vi "CAL_GCP_R.vi"(0 "Initialize":bool, 5 "R_ROLL":sgl, 7 "출력 클러스터 2":T1, 9 "B_ACC":sgl, 11 "R_power_raw":sgl) -> (3 "R_power_OK":bool, 4 "R_Ctrl_Start":bool, 6 "R_GCP":sgl, 8 "출력 클러스터":T1, 10 "R_Period":sgl, 15 "CAN":enum16{"stand", "init", "read"}(ring))   [LabVIEW 2019]
panel:
  out "R_power":sgl[](array[numeric])
  out "R_Run_OK":bool
  out "R_NUM":u32
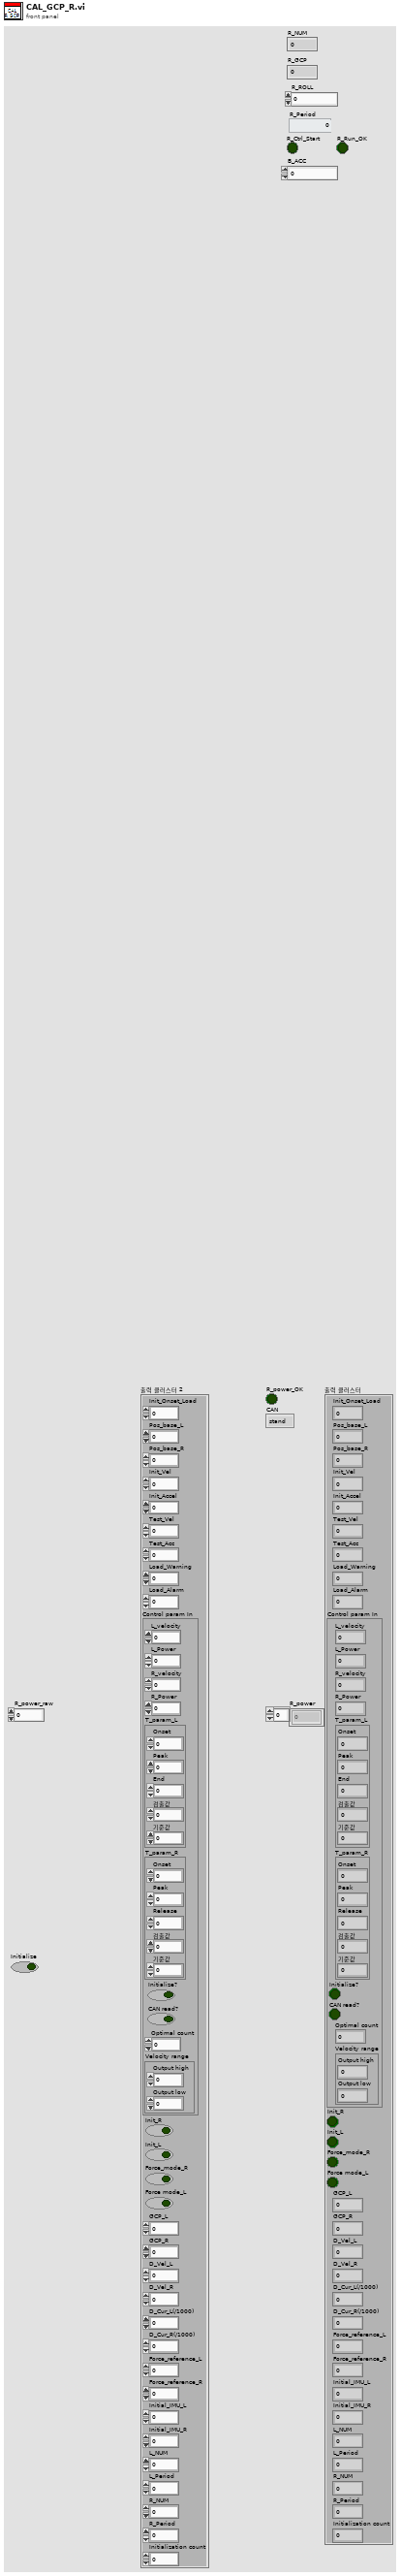
[diagram p1: front panel]
types:
  T1 = cluster{"Init_Onset_Load":sgl, "Pos_base_L":sgl, "Pos_base_R":sgl, "Init_Vel":i32, "Init_Accel":u32, "Test_Vel":i32, "Test_Acc":u32, "Load_Warning":sgl, "Load_Alarm":sgl, "Control param In":cluster{"L_velocity":u32, "L_Power":sgl, "R_velocity":u32, "R_Power":sgl, "T_param_L":cluster{"Onset":sgl, "Peak":sgl, "End":sgl, "검출값":sgl, "기준값":sgl}, "T_param_R":cluster{"Onset":sgl, "Peak":sgl, "Release":sgl, "검출값":sgl, "기준값":sgl}, "Initialize?":bool, "CAN read?":bool, "Optimal count":i32, "Velocity range":cluster{"Output high":dbl, "Output low":dbl}}, "Init_R":bool, "Init_L":bool, "Force_mode_R":bool, "Force mode_L":bool, "GCP_L":sgl, "GCP_R":sgl, "D_Vel_L":sgl, "D_Vel_R":sgl, "D_Cur_L(/1000)":sgl, "D_Cur_R(/1000)":sgl, "Force_reference_L":sgl, "Force_reference_R":sgl, "Initial_IMU_L":sgl, "Initial_IMU_R":sgl, "L_NUM":u32, "L_Period":i16, "R_NUM":u32, "R_Period":i16, "Initialization count":i32}
  T2 = enum16{"Init", "HF", "Cross", "HE", "Cross_E", "Init_F"}
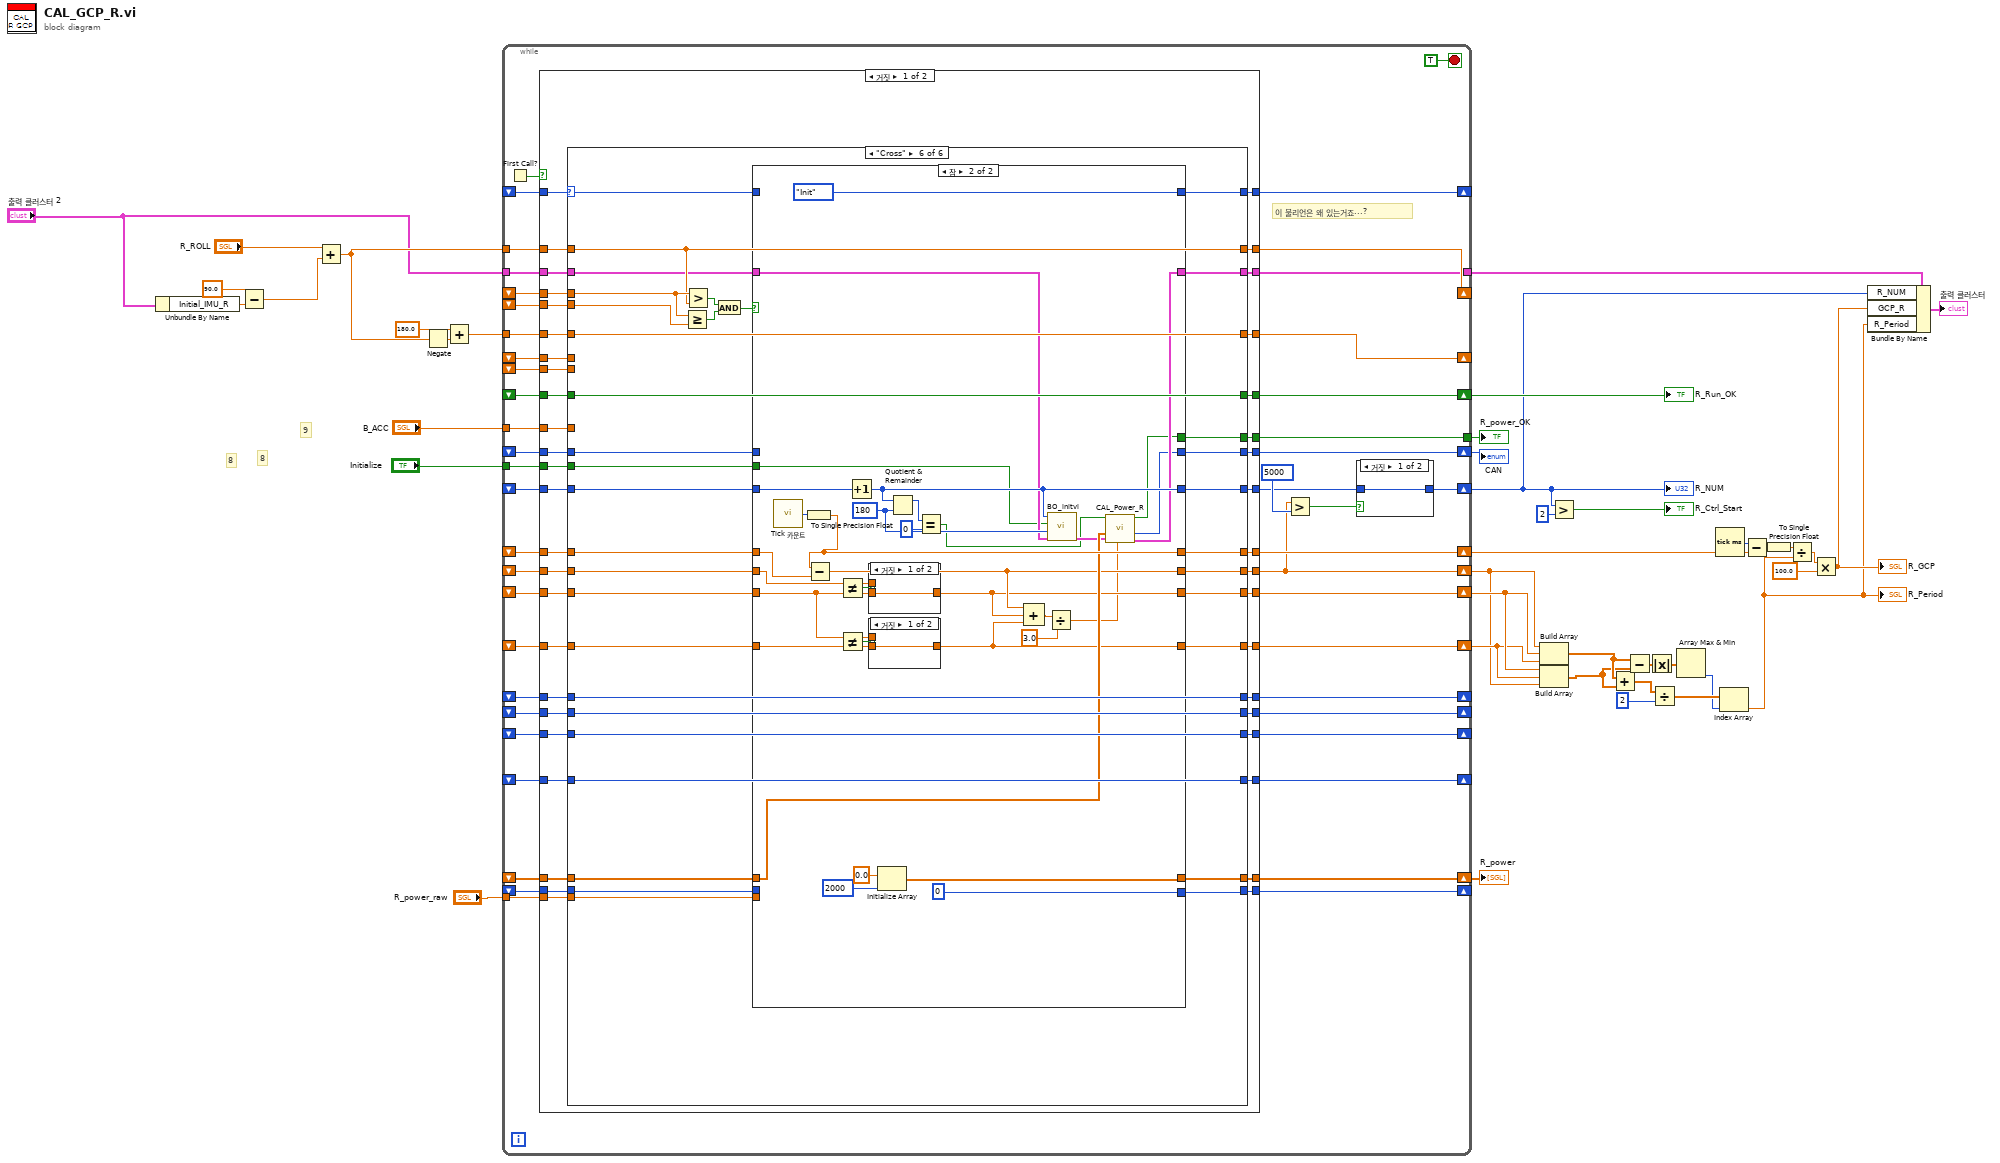
[diagram p0: block diagram]
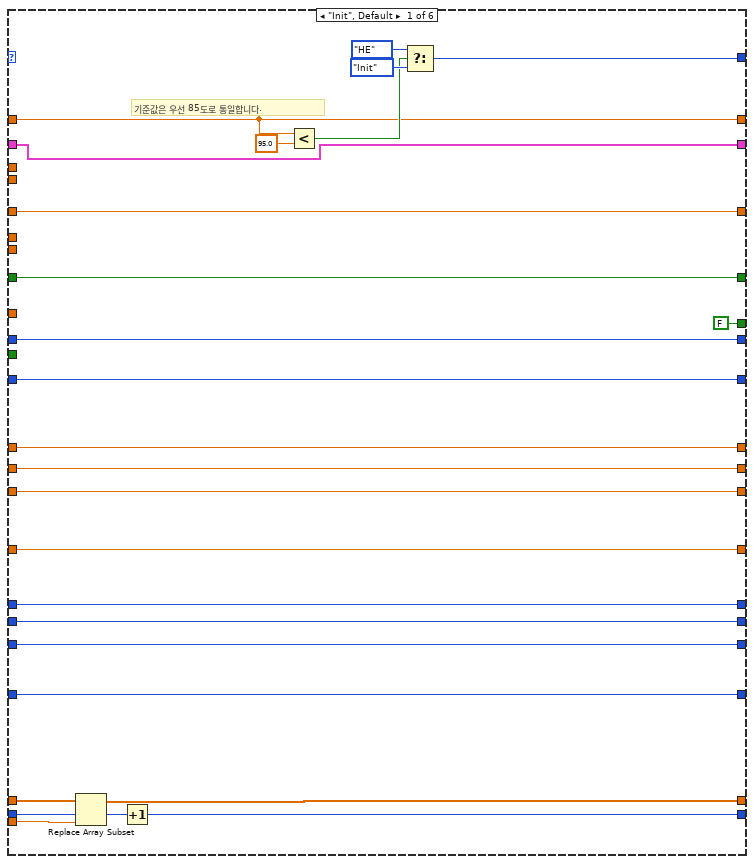
[diagram p2: hidden frame]
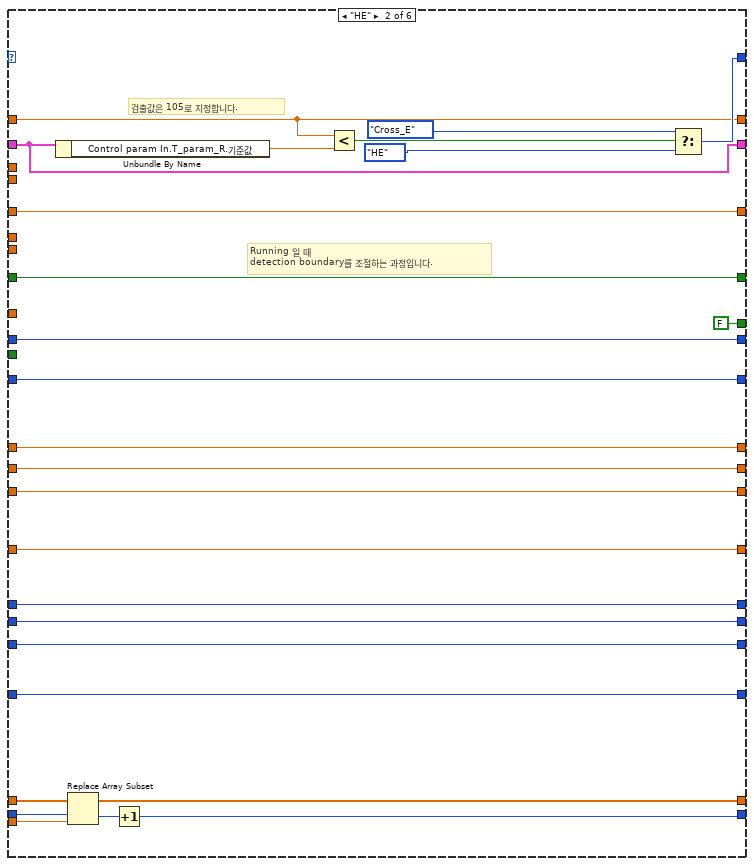
[diagram p3: hidden frame]
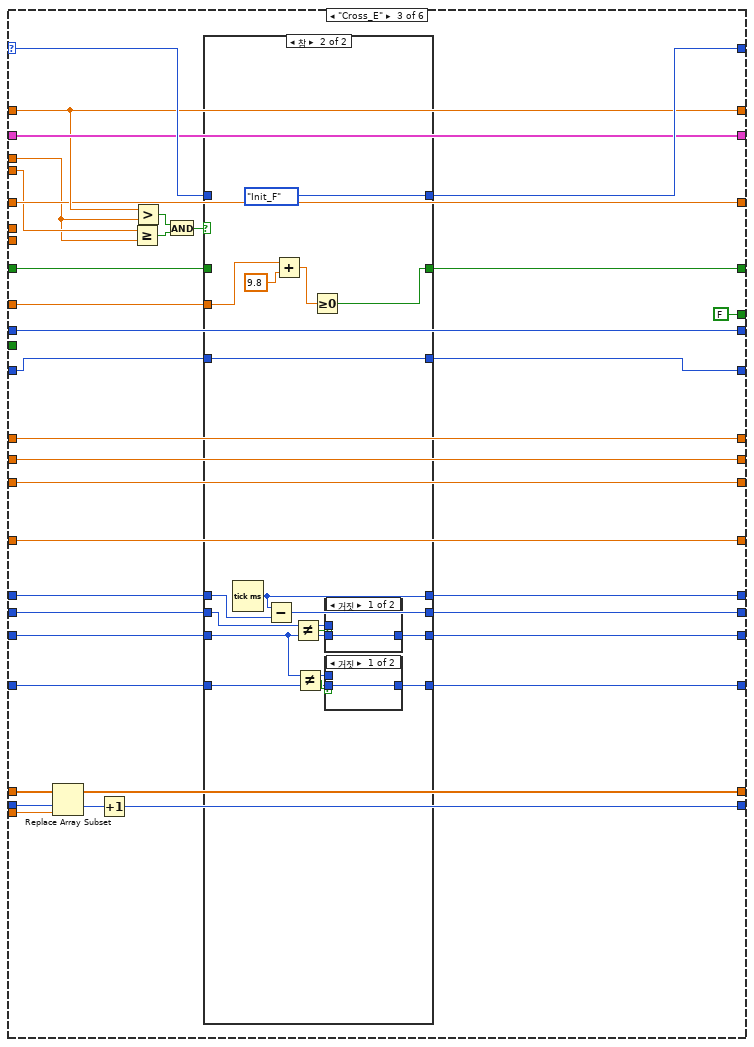
[diagram p4: hidden frame]
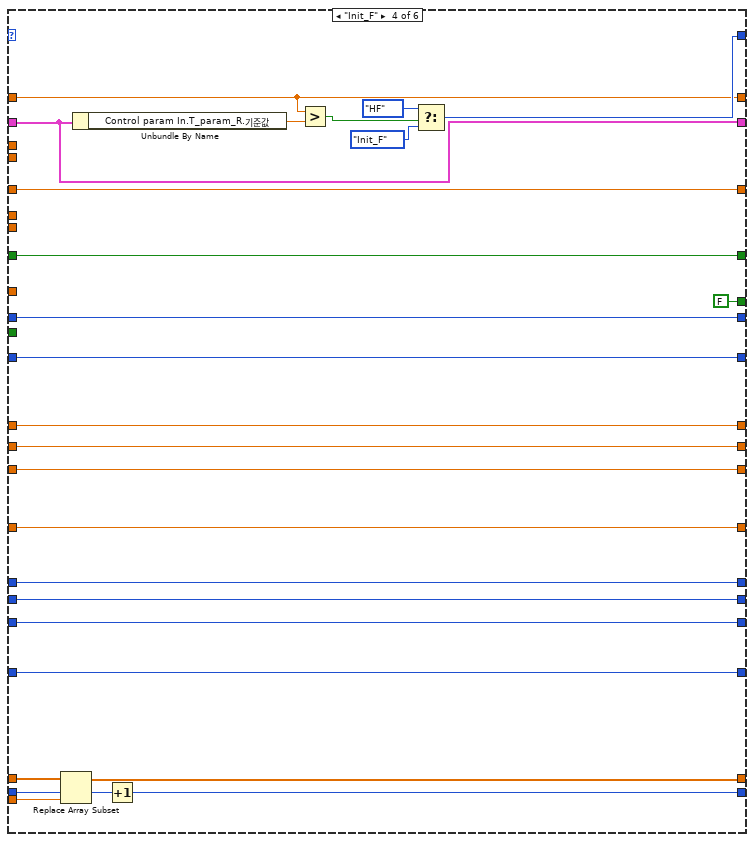
[diagram p8: hidden frame]
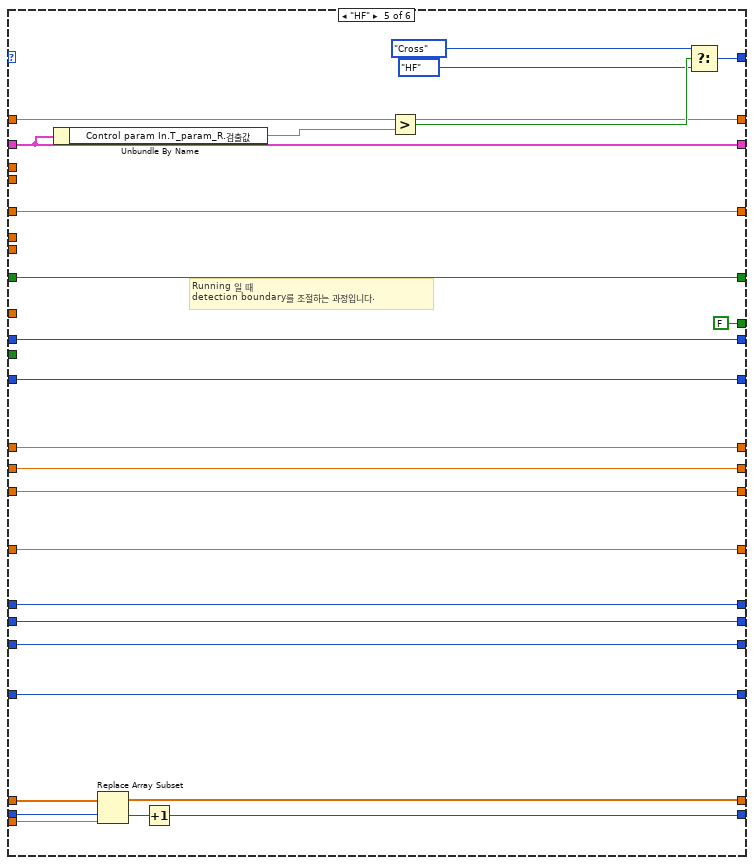
[diagram p9: hidden frame]
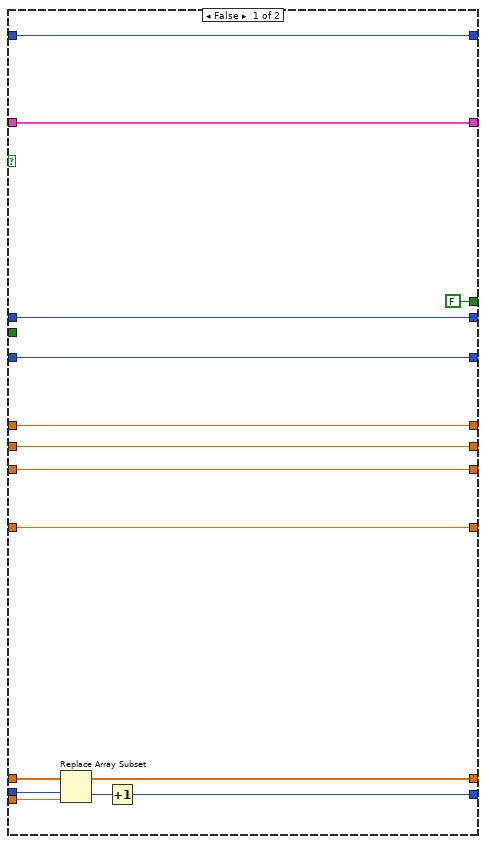
[diagram p10: hidden frame]
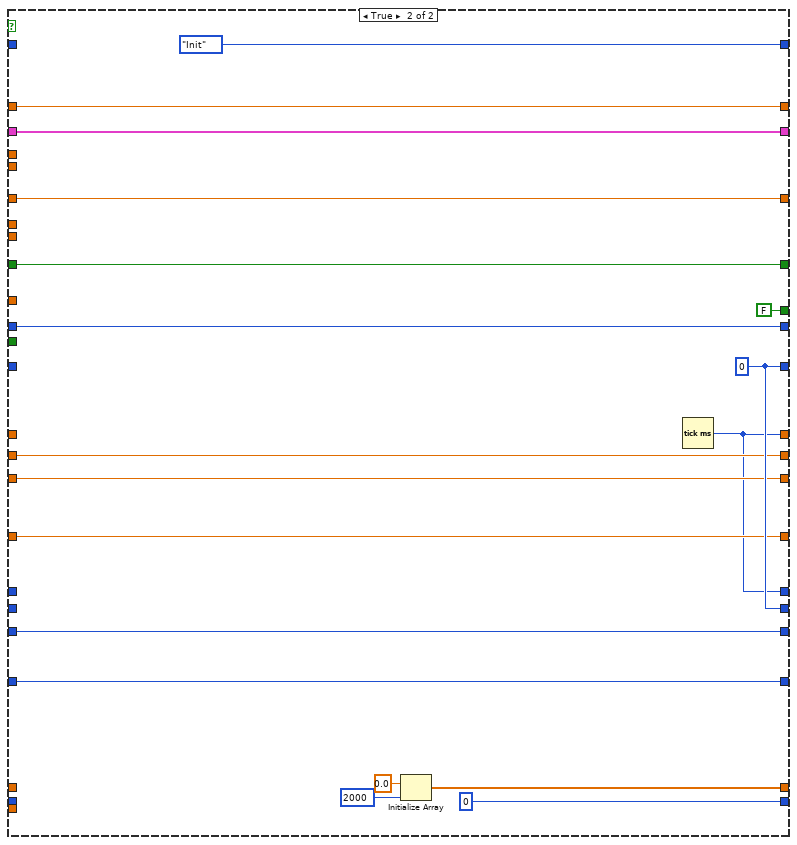
[diagram p13: hidden frame]
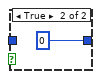
[diagram p14: hidden frame]
diagram:
  # "8"
  # "8"
  # "9"
  n1 = Unbundle By Name("출력 클러스터 2") -> ("Initial_IMU_R"=w5:sgl)
  n2 = Subtract(x=sgl 90.0, y=w5) -> (x-y=w1:sgl)
  n3 = Add(x="R_ROLL", y=w1) -> (x+y=w15:sgl)
  n4 = Negate(x=w15) -> (-x=w33:sgl)
  n5 = Add(x=sgl 180.0, y=w33) -> (x+y=w30:sgl)
  n6 = while {
    tunnel: w15 -> [w84]
    tunnel: "출력 클러스터 2" -> [w81]
    shift-right: [w53] -> _
    shift-left: _ -> [w52]
    shift-right: [w85] -> _
    shift-left: _ -> [w80]
    shift-left: _ -> [w79]
    shift-right: [w76] -> w11
    shift-left: _ -> [w83]
    shift-right: [w66] -> _
    shift-left: _ -> [w82]
    tunnel: w30 -> [w74]
    shift-right: [w73] -> _
    shift-left: _ -> [w72]
    shift-left: _ -> [w71]
    shift-right: [w70] -> w29
    shift-left: _ -> [w69]
    tunnel: "B_ACC" -> [w68]
    shift-right: [w65] -> _
    shift-left: _ -> [w67]
    shift-right: [w58] -> w22
    shift-left: _ -> [w57]
    shift-right: [w55] -> w21
    shift-left: _ -> [w56]
    shift-right: [w64] -> _
    shift-left: _ -> [w63]
    shift-right: [w61] -> _
    shift-left: _ -> [w62]
    shift-right: [w60] -> w28
    shift-left: _ -> [w59]
    shift-right: [w51] -> w20
    shift-left: _ -> [w54]
    shift-right: [w50] -> w13
    shift-left: _ -> [w48]
    shift-right: [w49] -> _
    shift-left: _ -> [w47]
    tunnel: "R_power_raw" -> [w46]
    tunnel: [w45] -> w12
    tunnel: "Initialize" -> [w44]
    tunnel: [w43] -> w7
    shift-right: [w42] -> w6
    shift-left: _ -> [w41]
    stop <- TRUE stop-if-true
    # "이 불리언은 왜 있는거죠...?"
    n7 = First Call?() -> (First Call?: T/F=w86:bool)
    n8 = case shown="거짓" w86 {
      tunnel: [w127 w393] -> w85
      tunnel: w84 -> [w128 w393]
      tunnel: w83 -> [w125 _]
      tunnel: [w126 w392] -> w75
      tunnel: [w123 w383] -> w66
      tunnel: [w122 w392] -> w65
      tunnel: w82 -> [w124 _]
      tunnel: w81 -> [w129 w378]
      tunnel: w80 -> [w121 _]
      tunnel: w79 -> [w120 _]
      tunnel: w74 -> [w119 w391]
      tunnel: [w118 w391] -> w73
      tunnel: w72 -> [w117 _]
      tunnel: w71 -> [w116 _]
      tunnel: [w114 w390] -> w70
      tunnel: w69 -> [w115 w390]
      tunnel: w68 -> [w113 _]
      tunnel: w67 -> [w112 _]
      tunnel: [w111 w389] -> w64
      tunnel: w63 -> [w110 w389]
      tunnel: w62 -> [w109 w388]
      tunnel: [w108 w388] -> w61
      tunnel: [w107 w383] -> w60
      tunnel: w59 -> [w106 _]
      tunnel: [w105 w387] -> w58
      tunnel: w57 -> [w104 w387]
      tunnel: w56 -> [w103 w386]
      tunnel: [w102 w386] -> w55
      tunnel: [w101 w385] -> w51
      tunnel: w54 -> [w100 w385]
      tunnel: [w98 T2."Init"] -> w53
      tunnel: w52 -> [w99 _]
      tunnel: [w94 w380] -> w50
      tunnel: [w93 0] -> w49
      tunnel: w48 -> [w97 _]
      tunnel: w47 -> [w96 _]
      tunnel: w46 -> [w95 _]
      tunnel: [w92 w378] -> w45
      tunnel: w44 -> [w91 _]
      tunnel: [w90 FALSE ("R_power_OK")] -> w43
      tunnel: [w89 w376] -> w42
      tunnel: w41 -> [w88 w376]
      frame False {
        n9 = case shown="\"Cross\"" w99 {
          selector: w99 -> [_ _ w213 _ _ w325]
          tunnel: w129 -> [w133 w158 w186 w241 w270 w296]
          tunnel: w128 -> [w131 w155 w183 w261 w289 w318]
          tunnel: [w131 w155 w183 w261 w289 w318] -> w127
          tunnel: [w154 w178 w211 w258 w288 w320] -> w126
          tunnel: w125 -> [w154 w178 w212 w258 w288 w321]
          tunnel: w124 -> [w153 w177 w209 w257 w287 w313]
          tunnel: [w153 w177 w210 w257 w287 w313] -> w123
          tunnel: [w150 w176 w208 w256 w286 w316] -> w122
          tunnel: w121 -> [_ _ w180 _ _ w319]
          tunnel: w120 -> [_ _ w181 _ _ w324]
          tunnel: w119 -> [w152 w172 w182 w260 w282 w310]
          tunnel: [w152 w172 w182 w260 w282 w310] -> w118
          tunnel: w117 -> [_ _ _ _ _ _]
          tunnel: w116 -> [_ _ _ _ _ _]
          tunnel: w115 -> [w151 w169 w207 w259 w267 w309]
          tunnel: [w151 w169 w206 w259 w267 w309] -> w114
          tunnel: w113 -> [_ _ w205 _ _ _]
          tunnel: w112 -> [w150 w176 w193 w256 w286 w316]
          tunnel: [w149 w175 w201 w254 w285 w315] -> w111
          tunnel: w110 -> [w149 w175 w192 w254 w285 w315]
          tunnel: w109 -> [w148 w174 w200 w253 w284 w314]
          tunnel: [w148 w174 w199 w253 w284 w314] -> w108
          tunnel: [w147 w173 w198 w255 w283 w312] -> w107
          tunnel: w106 -> [w147 w173 w198 w255 w283 w311]
          tunnel: [w146 w171 w196 w251 w281 w308] -> w105
          tunnel: w104 -> [w146 w171 w196 w251 w281 w307]
          tunnel: w103 -> [w145 w170 w197 w250 w280 w306]
          tunnel: [w145 w170 w197 w250 w280 w305] -> w102
          tunnel: [w144 w168 w195 w252 w279 w304] -> w101
          tunnel: w100 -> [w144 w168 w195 w252 w279 w303]
          tunnel: [w143 w165 w194 w262 w276 w302] -> w98
          tunnel: w97 -> [w139 w164 w191 w248 w275 w301]
          tunnel: w96 -> [w136 w163 w190 w247 w274 w300]
          tunnel: w95 -> [w138 w162 w189 w246 w273 w299]
          tunnel: [w137 w161 w187 w245 w272 w297] -> w94
          tunnel: [w135 w160 w188 w244 w271 w298] -> w93
          tunnel: [w133 w158 w186 w241 w270 w295] -> w92
          tunnel: w91 -> [_ _ _ _ _ w294]
          tunnel: [FALSE ("R_power_OK") FALSE ("R_power_OK") FALSE ("R_power_OK") FALSE ("R_power_OK") FALSE ("R_power_OK") w293] -> w90
          tunnel: [w132 w157 w184 w242 w268 w292] -> w89
          tunnel: w88 -> [w132 w157 w184 w242 w268 w291]
          frame "Init", Default {
            # "기준값은 우선 85도로 통일합니다."
            n10 = Replace Array Subset(array=w139, new element=w138, index=w136) -> (w137:sgl[])
            n11 = Increment(x=w136) -> (x+1=w135:i32)
            n12 = Less?(x=w131, y=sgl 95.0) -> (x < y?=w140:bool)
            n13 = Select(t=T2."HE", s=w140, f=T2."Init") -> (s? t:f=w143:T2)
          }
          frame "HE" {
            # "Running 일 때 \ndetection boundary를 조절하는 과정입니다."
            # "검출값은 105로 지정합니다."
            n14 = Unbundle By Name(w158) -> ("Control param In.T_param_R.기준값"=w156:sgl)
            n15 = Replace Array Subset(array=w164, new element=w162, index=w163) -> (w161:sgl[])
            n16 = Increment(x=w163) -> (x+1=w160:i32)
            n17 = Less?(x=w155, y=w156) -> (x < y?=w179:bool)
            n18 = Select(t=T2."Cross_E", s=w179, f=T2."HE") -> (s? t:f=w165:T2)
          }
          frame "Cross_E" {
            n19 = Replace Array Subset(array=w191, new element=w189, index=w190) -> (w187:sgl[])
            n20 = Increment(x=w190) -> (x+1=w188:i32)
            n21 = Greater Or Equal?(x=w181, y=w180) -> (x >= y?=w204:bool)
            n22 = Greater?(x=w183, y=w180) -> (0:w203:bool)
            n23 = And(x=w203, y=w204) -> (x .and. y?=w202:bool)
            n24 = case shown="참" w202 {
              tunnel: w213 -> [w218 _]
              tunnel: [w218 T2."Init_F"] -> w194
              tunnel: w212 -> [w219 w227]
              tunnel: [w219 w227] -> w211
              tunnel: w209 -> [w220 w236]
              tunnel: [w215 w226] -> w208
              tunnel: [w220 w235] -> w210
              tunnel: w207 -> [w217 _]
              tunnel: [w217 w232] -> w206
              tunnel: w205 -> [_ w221]
              tunnel: [w214 w231] -> w201
              tunnel: w200 -> [w216 w230]
              tunnel: [w216 w229] -> w199
              tunnel: w193 -> [w215 w225]
              tunnel: w192 -> [w214 w224]
              frame False {
              }
              frame True {
                n25 = Tick Count (ms)() -> (millisecond timer value=w235:u32)
                n26 = Subtract(x=w235, y=w236) -> (x-y=w226:u32)
                n27 = Add(x=w221, y=9.8) -> (x+y=w222:dbl)
                n28 = Not Equal?(x=w225, y=w224) -> (x != y?=w234:bool)
                n29 = Not Equal?(x=w224, y=w230) -> (x != y?=w233:bool)
                n30 = Greater Or Equal To 0?(x=w222) -> (x >= 0?=w232:bool)
                n31 = case shown="거짓" w234 {
                  tunnel: [w239 w240] -> w231
                  tunnel: w225 -> [_ w240]
                  tunnel: w224 -> [w239 _]
                  frame False {
                  }
                  frame True {
                  }
                }
                n32 = case shown="거짓" w233 {
                  tunnel: w224 -> [_ w238]
                  tunnel: w230 -> [w237 _]
                  tunnel: [w237 w238] -> w229
                  frame False {
                  }
                  frame True {
                  }
                }
              }
            }
          }
          frame "Init_F" {
            n33 = Replace Array Subset(array=w248, new element=w246, index=w247) -> (w245:sgl[])
            n34 = Unbundle By Name(w241) -> ("Control param In.T_param_R.기준값"=w265:sgl)
            n35 = Increment(x=w247) -> (x+1=w244:i32)
            n36 = Greater?(x=w261, y=w265) -> (0:w249:bool)
            n37 = Select(t=T2."HF", s=w249, f=T2."Init_F") -> (s? t:f=w262:T2)
          }
          frame "HF" {
            # "Running 일 때 \ndetection boundary를 조절하는 과정입니다."
            n38 = Unbundle By Name(w270) -> ("Control param In.T_param_R.검출값"=w266:sgl)
            n39 = Replace Array Subset(array=w275, new element=w273, index=w274) -> (w272:sgl[])
            n40 = Increment(x=w274) -> (x+1=w271:i32)
            n41 = Greater?(x=w289, y=w266) -> (0:w290:bool)
            n42 = Select(t=T2."Cross", s=w290, f=T2."HF") -> (s? t:f=w276:T2)
          }
          frame "Cross" {
            n43 = Greater Or Equal?(x=w319, y=w324) -> (x >= y?=w323:bool)
            n44 = Greater?(x=w319, y=w318) -> (0:w317:bool)
            n45 = And(x=w317, y=w323) -> (x .and. y?=w322:bool)
            n46 = case shown="참" w322 {
              tunnel: w325 -> [w338 _]
              tunnel: [w338 T2."Init"] -> w302
              tunnel: w321 -> [w339 w366]
              tunnel: [w339 w356] -> w320
              tunnel: [w337 w362] -> w312
              tunnel: w311 -> [w337 w369]
              tunnel: [w336 w347] -> w308
              tunnel: w307 -> [w336 w364]
              tunnel: w306 -> [w335 w368]
              tunnel: [w335 w346] -> w305
              tunnel: [w334 w348] -> w304
              tunnel: w303 -> [w334 w365]
              tunnel: w301 -> [w333 w353]
              tunnel: w300 -> [w332 _]
              tunnel: w299 -> [w331 _]
              tunnel: [w330 0] -> w298
              tunnel: [w329 w358] -> w297
              tunnel: w296 -> [w326 w354]
              tunnel: [w326 w351] -> w295
              tunnel: w294 -> [_ w341]
              tunnel: [FALSE ("R_power_OK") w340] -> w293
              tunnel: [w327 w350] -> w292
              tunnel: w291 -> [w327 _]
              frame False {
                n47 = Replace Array Subset(array=w333, new element=w331, index=w332) -> (w329:sgl[])
                n48 = Increment(x=w332) -> (x+1=w330:i32)
              }
              frame True {
                w355 = u32 180 ("y")
                n49 = call "Tick 카운트"() -> ("Tick Count(mSec)"=w363:u32)
                n50 = To Single Precision Float(number=w363) -> (single precision float=w362:sgl)
                n51 = Subtract(x=w362, y=w369) -> (x-y=w348:sgl)
                n52 = Not Equal?(x=w365, y=w364) -> (x != y?=w371:bool)
                n53 = Not Equal?(x=w364, y=w368) -> (x != y?=w370:bool)
                n54 = Increment(x=w366) -> (x+1=w356:u32)
                n55 = case shown="거짓" w371 {
                  tunnel: w365 -> [_ w375]
                  tunnel: [w374 w375] -> w347
                  tunnel: w364 -> [w374 _]
                  frame False {
                  }
                  frame True {
                  }
                }
                n56 = case shown="거짓" w370 {
                  tunnel: w364 -> [_ w373]
                  tunnel: w368 -> [w372 _]
                  tunnel: [w372 w373] -> w346
                  frame False {
                  }
                  frame True {
                  }
                }
                n57 = Initialize Array(sgl 0.0 ("원소"), 2000 ("차원 크기")) -> (w358:sgl[])
                n58 = Quotient & Remainder(x=w356, y=w355) -> (x-y*floor(x/y)=w357:u32)  [unwired: 1 out]
                n59 = Equal?(x=w357, y=u32 0) -> (x = y?=w349:bool)
                n60 = Compound Arithmetic op=ADD(w348, w347, w346) -> (w345:sgl)
                n61 = Divide(x=w345, y=sgl 3.0) -> (x/y=w343:sgl)
                n62 = call "BO_initvi.vi"("출력 클러스터 2"=w354, "Stride number"=w355, "Initialize"=w341, "R_NUM"=w356) -> ("출력 클러스터 3"=w352:T1)  [unwired: 7 in]
                n63 = call "CAL_Power_R.vi"("Stride?"=w349, "Positive Power"=w353, "출력 클러스터 2"=w352, "Period_R"=w343) -> ("R_power_OK"=w340:bool, "CAN"=w350:enum16{"stand", "init", "read"}, "출력 클러스터 3"=w351:T1)  [unwired: 4 in]
              }
            }
          }
        }
      }
      frame True {
        w392 = u32 0
        n64 = Initialize Array(sgl 0.0 ("원소"), 2000 ("차원 크기")) -> (w380:sgl[])
        n65 = Tick Count (ms)() -> (millisecond timer value=w383:u32)
      }
    }
    n66 = Greater?(x=w51, y=u32 5000) -> (0:w77:bool)
    n67 = case shown="거짓" w77 {
      tunnel: [w394 u32 0] -> w76
      tunnel: w75 -> [w394 _]
      frame False {
      }
      frame True {
      }
    }
  }
  "R_NUM" <- w11
  "R_Run_OK" <- w29
  "R_power" <- w13
  "R_power_OK" <- w7
  "CAN" <- w6
  n68 = Build Array(w20, w22, w21) -> (w19:sgl[])
  n69 = Build Array(w22, w21, w20) -> (w18:sgl[])
  n70 = Greater?(x=w11, y=u32 2) -> (0:→"R_Ctrl_Start":bool)
  n71 = Add(x=w19, y=w18) -> (x+y=w25:sgl[])
  n72 = Subtract ("빼기")(x=w19, y=w18) -> (x-y=w27:sgl[])
  n73 = Absolute Value(x=w27) -> (abs(x)=w26:sgl[])
  n74 = Divide ("나누기")(x=w25, y=2) -> (x/y=w23:sgl[])
  n75 = Array Max & Min(array=w26) -> (min index (indices)=w17:i32)  [unwired: 3 out]
  n76 = Tick Count (ms)() -> (millisecond timer value=w36:u32)
  n77 = Index Array(array=w23, index=w17) -> (element=w9:sgl)
  "R_Period" <- w9
  n78 = Subtract(x=w36, y=w28) -> (x-y=w35:sgl)
  n79 = To Single Precision Float(number=w35) -> (single precision float=w32:sgl)
  n80 = Divide(x=w32, y=w9) -> (x/y=w38:sgl)
  n81 = Multiply(x=w38, y=sgl 100.0) -> (x*y=w10:sgl)
  "R_GCP" <- w10
  n82 = Bundle By Name(cluster=w12, "R_NUM"=w11, "GCP_R"=w10, "R_Period"=w9) -> (→"출력 클러스터":T1)
